vi "AnalogDemultiplexerV3_NI5771.vi"() -> ()   [LabVIEW 2012]
uses:
  <vilib>/Platform/TimedLoop/XDataNode/timing_clust.ctl
  <vilib>/Platform/TimedLoop/XDataNode/nitl_modes.ctl
  <vilib>/Platform/TimedLoop/XDataNode/wakeup.ctl
  <vilib>/rvi/FIFO/Fifo_Resource/nirvififoEmulationSetSize.vi
  <vilib>/rvi/DataTransferAndStorage/Container/Common/niFpgaContainerGetUniqueNameForEmu.vi
  <vilib>/rvi/eio/common/nirviEmuTemplateMethod_errors.vi
  <vilib>/rvi/Emulation/niFpgaSctlEmulationRegisterWithScheduler.vi
  <vilib>/rvi/errors/niFpgaSetErrorForExecOnDevCompSimple.vi
  <vilib>/rvi/eio/common/nirviEmuReportErrorAndStop.vi
  <vilib>/rvi/Emulation/niFpgaSctlEmulationFifoFullMgr.vi
  <vilib>/rvi/Emulation/niFpgaSctlEmulationResourceMgr.vi
  <vilib>/rvi/Emulation/niFpgaSctlEmulationScheduler.vi
  <vilib>/rvi/interface/RandomDataEmulation/nirviRandomDataFPGAFIFO.vi
  <vilib>/rvi/interface/RandomDataEmulation/niFpgaRandomDataHandleErrors.vi
  <vilib>/rvi/Emulation/niFpgaSctlEmulationGlobalWrite.vi
  <vilib>/Platform/TimedLoop/XDataNode/XDataNode.xnode
  <vilib>/rvi/DataTransferAndStorage/Container/XNode/niFpgaContainer.xnode
  <vilib>/rvi/FIFO/Fifo_Resource/nirvififoEmulationClear.vi
  <vilib>/eio/EIONode/EIONode.xnode
  <vilib>/rvi/FIFO/Fifo_Resource/nirvififoEmulationWrite.vi
  <vilib>/rvi/FIFO/Fifo_Resource/nirvififoEmulationRead.vi
  <vilib>/rvi/interface/RandomDataEmulation/nirviRandomDataFpgaReadWriteTemplate.vi
  <vilib>/Platform/TimedLoop/XDataNode/XDNodeRunTimeDep.lvlib
panel:
  out "Laser HIGH count per pixel":u16
  out "ToHostA2FIFO Overflow":bool
  out "ToHostA1FIFO Overflow":bool
  out "Pixel counter A2":u32
  out "Pixel counter A1":u32
  out "InterloopFIFO Overflow":bool
  in  "BaselineU8 Ch2":u8
  in  "BaselineU8 Ch1":u8
  out "InterloopFIFO timeout":bool
  in  "Clear Interloop FIFO":bool
  out "Acquiring":bool
  in  "Wait for trigger":bool
  in  "Acquire":bool
  in  "Requested pixels A2":u32=100000 caption="Requested pixels"
  in  "Acquire continuously":bool=TRUE
  in  "Requested pixels A1":u32=100000 caption="Requested pixels"
  in  "Samples per pixel":u16=10000 caption="Samples per pixel Acq"
  out "IO Module\\AI Over Range":bool
  in  "User Command Commit":bool
  in  "User Command":u8
  out "User Command Idle":bool
  out "User Command Status":u8
  in  "User Data 0":u16
  in  "User Data 1":u8
  out "PLL Locked":bool
  out "User Error":bool
  out "Configured?":bool
  # "5771 IO module configuration"
  # "Analog demultiplexer V3"
  # "Acquisition control"
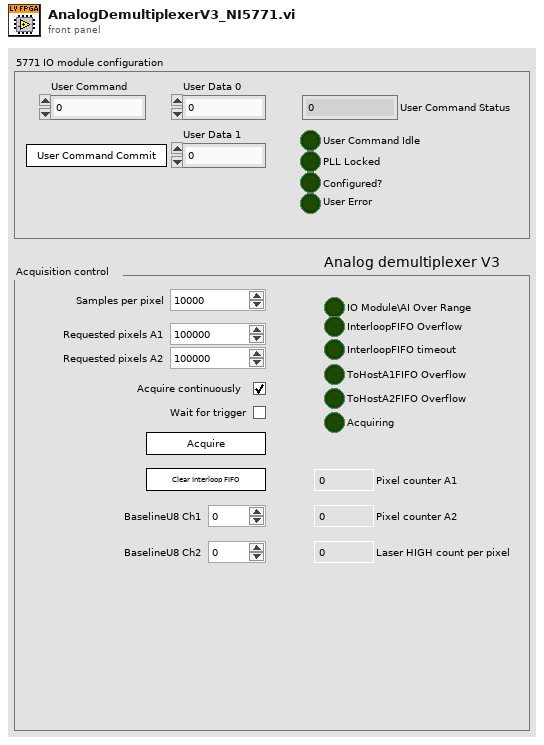
[diagram p1: front panel]
types:
  T1 = typedef "XDNodeRunTimeDep.lvlib/timing_clust.ctl" = cluster{"Expected End [f-1]":u64, "Actual End [f-1]":u64, "Finished Late? [f-1]":bool, "Expected End [i-1]":u64, "Actual End [i-1]":u64, "Finished Late? [i-1]":bool, "Expected Start [i]":u64, "Actual Start [i]":u64, "Expected Start [f]":u64, "Actual Start [f]":u64, "Source Name":string, "Structure Name":string, "Period":i64, "Deadline":i64, "Offset":i64, "Start":i64, "Priority":i32, "Timeout":i32, "Mode":T2, "Wakeup Reason":T3, "Error":errorcluster, "Source Type":string, "Secondary Source Type":string, "Global End Time":u64, "Global Start Time":u64, "Frame Duration":u64, "Iteration Duration":u64, "Assigned CPU":i32, "I/O Scan Engine Mode":u32}
  T2 = typedef "XDNodeRunTimeDep.lvlib/nitl_modes.ctl" = enum32{"No Change", "Process missed periods, maintain original phase", "Discard missed periods, maintain original phase", "Process missed periods, ignore original phase", "Discard missed periods, ignore original phase"}
  T3 = typedef "XDNodeRunTimeDep.lvlib/wakeup.ctl" = enum32{"Normal", "Aborted", "Asynchronous wakeup", "Timing source error", "Timed loop error", "Timeout"}
  T4 = cluster{"IO Module\\AI 0 Data N-7":u8, "IO Module\\AI 0 Data N-6":u8, "IO Module\\AI 0 Data N-5":u8, "IO Module\\AI 0 Data N-4":u8, "IO Module\\AI 0 Data N-3":u8, "IO Module\\AI 0 Data N-2":u8, "IO Module\\AI 0 Data N-1":u8, "IO Module\\AI 0 Data N":u8, "IO Module\\Synchronous Trigger Input":u8}
  T5 = cluster{"IO Module\\AI 1 Data N-7":u8, "IO Module\\AI 1 Data N-6":u8, "IO Module\\AI 1 Data N-5":u8, "IO Module\\AI 1 Data N-4":u8, "IO Module\\AI 1 Data N-3":u8, "IO Module\\AI 1 Data N-2":u8, "IO Module\\AI 1 Data N-1":u8, "IO Module\\AI 1 Data N":u8, "IO Module\\Synchronous Trigger Input":u8}
  T6 = cluster{"A1 Ch1":u32, "A1 Ch2":u32, "A2 Ch1":u32, "A2 Ch2":u32}
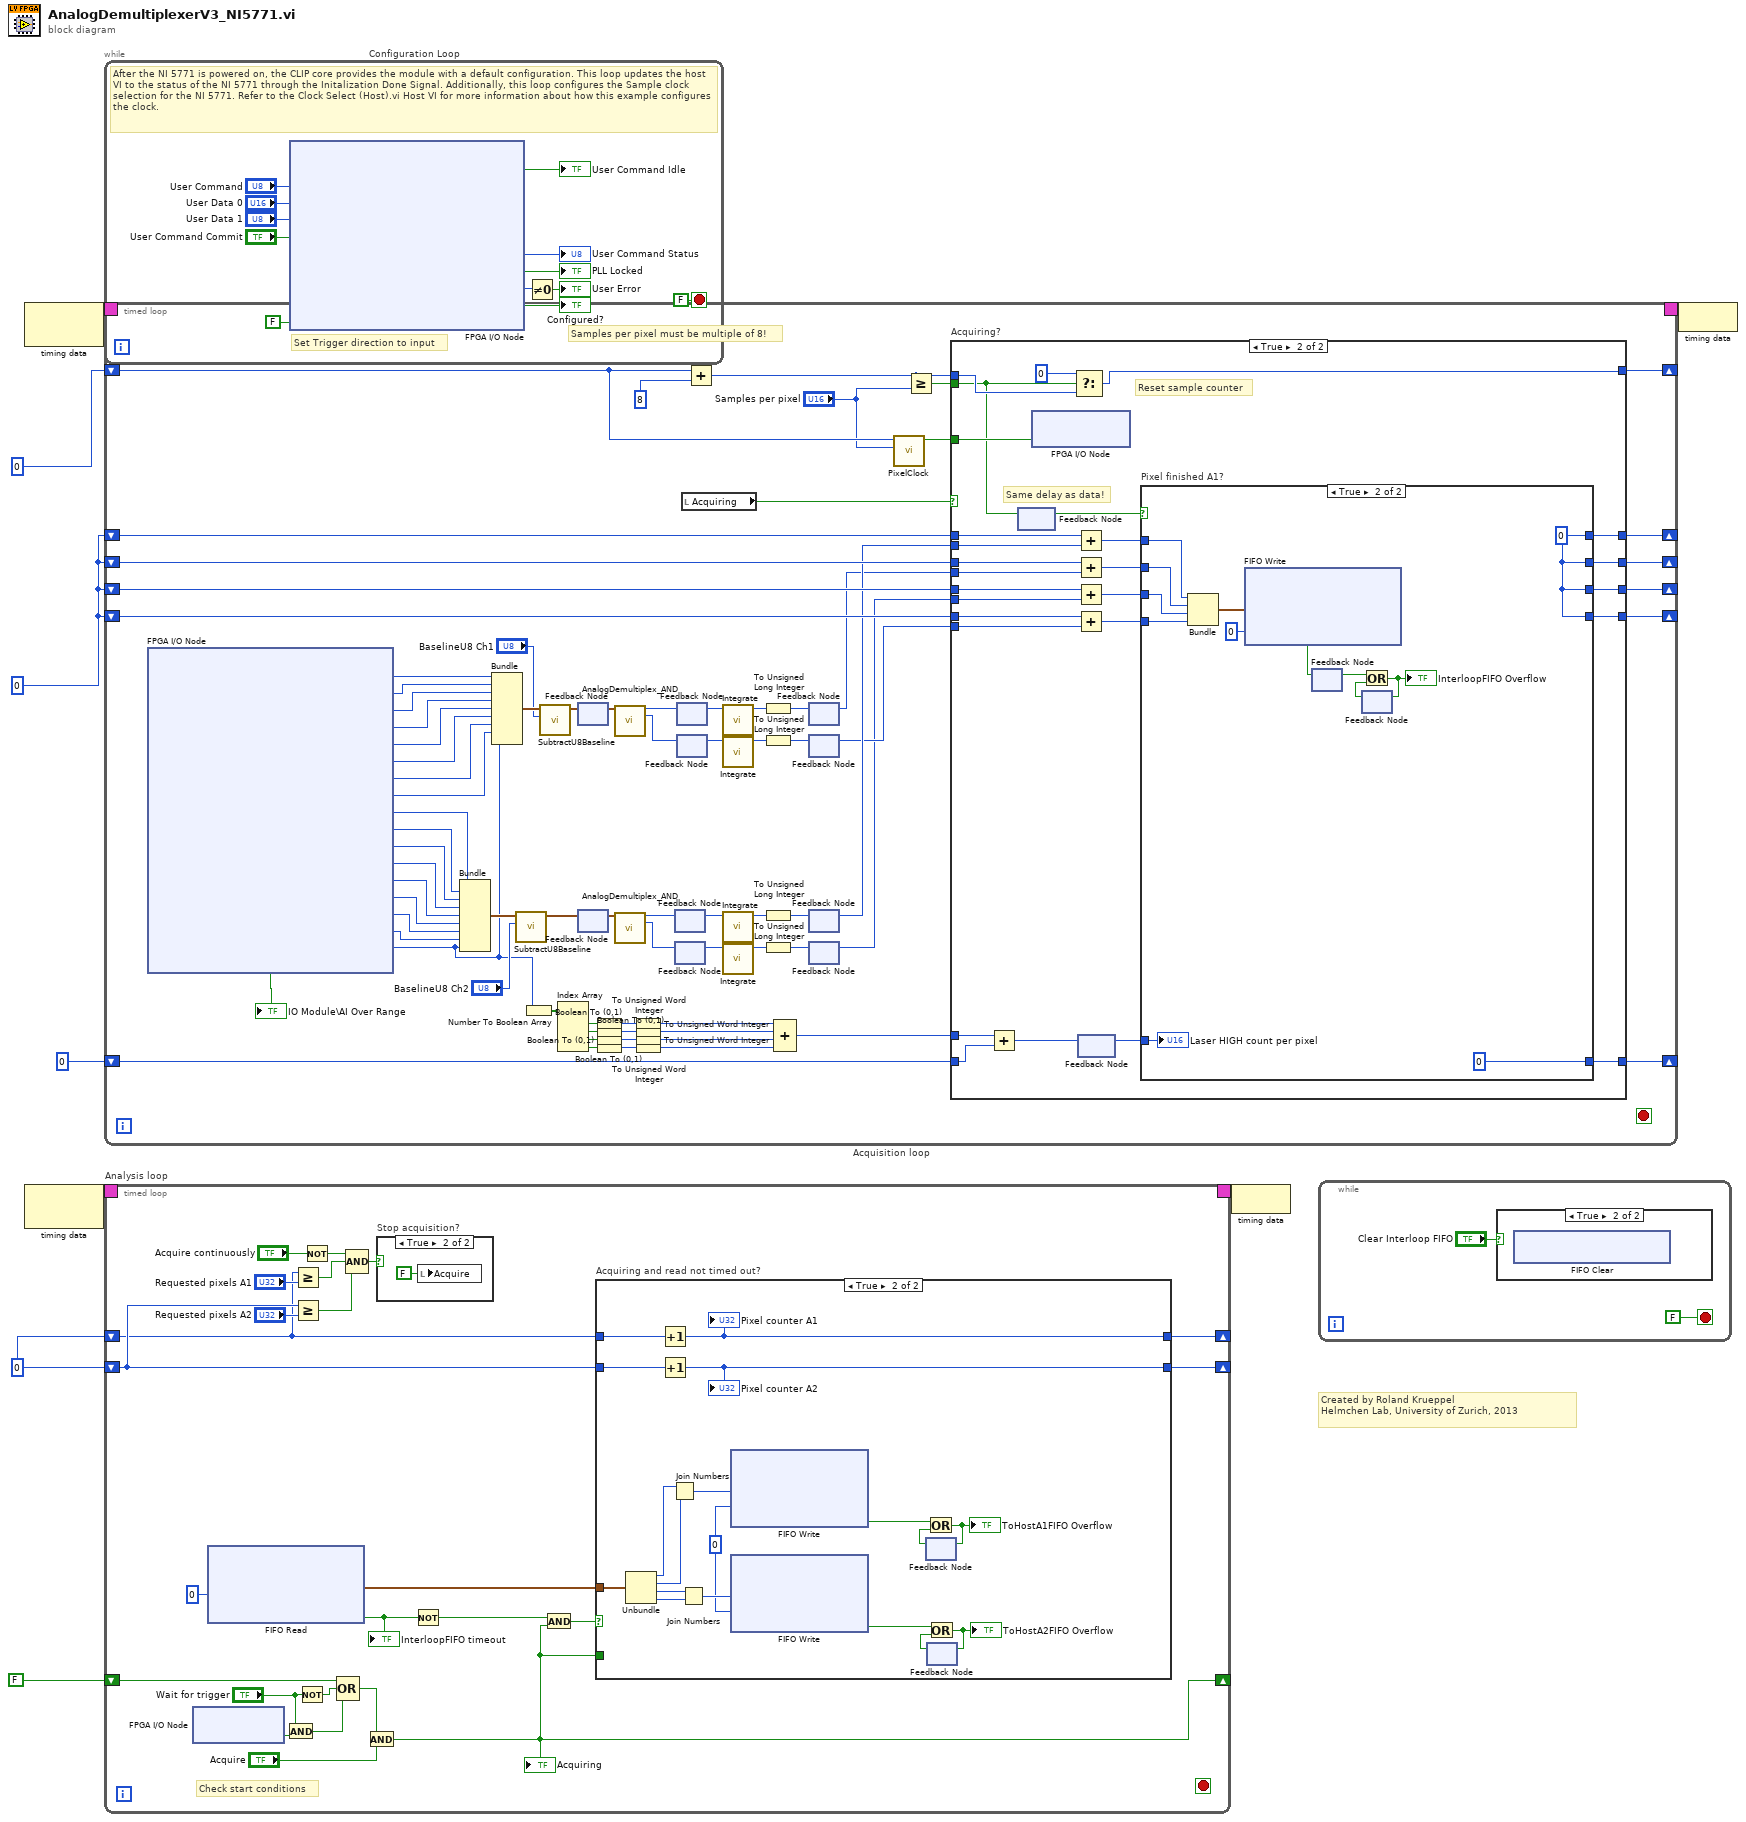
[diagram p0: block diagram]
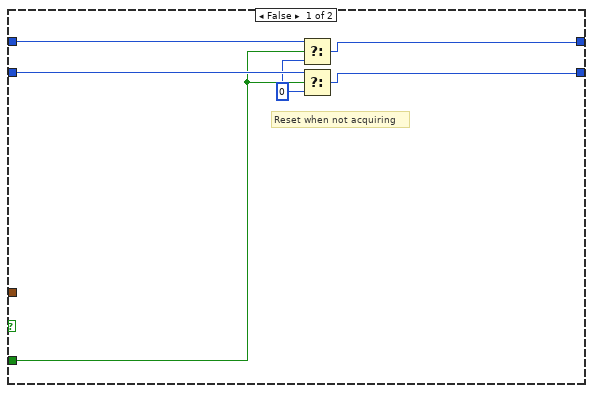
[diagram p3: hidden frame]
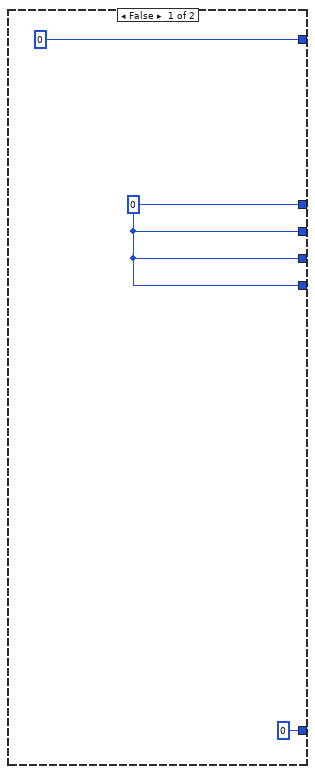
[diagram p5: hidden frame]
diagram:
  w2 = u32 0
  w3 = u32 0 ("Integrator out")
  # "Created by Roland Krueppel\nHelmchen Lab, University of Zurich, 2013"
  n1 = node-c288() -> (w9:T1)  [unwired: 1 in]
  n2 = node-c288() -> (w7:T1)  [unwired: 1 in]
  n3 = while "Configuration Loop" {
    stop <- FALSE stop-if-true
    # "Set Trigger direction to input"
    # "After the NI 5771 is powered on, the CLIP core provides the module with a default configuration. This loop updates the host VI to the status of the NI 5771 through the Initalization Done Signal. Additionally, this loop configures the Sample clock selection for the NI 5771. Refer to the Clock Select (Host).vi Host VI for more information about how this example configures the clock."
    n4 = xnode "FPGA I/O Node"("IO Module\\User Command"="User Command", "IO Module\\User Data 0"="User Data 0", "IO Module\\User Data 1"="User Data 1", "IO Module\\User Command Commit"="User Command Commit", "IO Module\\Trigger WE"=FALSE ("IO Module\\Trigger WE")) -> ("IO Module\\User Command Idle"=→"User Command Idle":bool, "IO Module\\User Command Status"=→"User Command Status":u8, "IO Module\\PLL Locked"=→"PLL Locked":bool, "IO Module\\User Error"=w14:u8, "IO Module\\Initialization Done"=→"Configured?":bool)  [unwired: 10 in, 10 out]
    n5 = Not Equal To 0?(x=w14) -> (x != 0?=→"User Error":bool)
  }
  n6 = timed-loop "Acquisition loop" {
    timing: w9 -> [_]
    timing-out: [_] -> w8
    shift-right: [w83] -> _
    shift-left: u16 0 -> [w70]
    shift-right: [w40] -> _
    shift-left: w2 -> [w49]
    shift-right: [w39] -> _
    shift-left: w2 -> [w48]
    shift-right: [w41] -> _
    shift-left: w2 -> [w50]
    shift-right: [w42] -> _
    shift-left: w2 -> [w51]
    shift-right: [w22] -> _
    shift-left: u16 0 -> [w23]
    stop <- _ stop-if-true
    # "Samples per pixel must be multiple of 8!"
    n7 = xnode "FPGA I/O Node"() -> ("IO Module\\AI 1 Data N-7"=w91:u8, "IO Module\\AI 1 Data N-6"=w90:u8, "IO Module\\AI 1 Data N-5"=w89:u8, "IO Module\\AI 1 Data N-4"=w88:u8, "IO Module\\AI 1 Data N-3"=w87:u8, "IO Module\\AI 1 Data N-2"=w86:u8, "IO Module\\AI 1 Data N-1"=w85:u8, "IO Module\\AI 1 Data N"=w84:u8, "IO Module\\AI 0 Data N-7"=w92:u8, "IO Module\\AI 0 Data N-6"=w93:u8, "IO Module\\AI 0 Data N-5"=w94:u8, "IO Module\\AI 0 Data N-4"=w95:u8, "IO Module\\AI 0 Data N-3"=w96:u8, "IO Module\\AI 0 Data N-2"=w97:u8, "IO Module\\AI 0 Data N-1"=w98:u8, "IO Module\\AI 0 Data N"=w99:u8, "IO Module\\Synchronous Trigger Input"=w38:u8, "IO Module\\AI Over Range"=→"IO Module\\AI Over Range":bool)  [unwired: 18 in, 18 out]
    n8 = Bundle("IO Module\\AI 0 Data N-7"=w92, "IO Module\\AI 0 Data N-6"=w93, "IO Module\\AI 0 Data N-5"=w94, "IO Module\\AI 0 Data N-4"=w95, "IO Module\\AI 0 Data N-3"=w96, "IO Module\\AI 0 Data N-2"=w97, "IO Module\\AI 0 Data N-1"=w98, "IO Module\\AI 0 Data N"=w99, "IO Module\\Synchronous Trigger Input"=w38) -> (w74:T4)  [unwired: 1 in]
    n9 = Bundle("IO Module\\AI 1 Data N-7"=w91, "IO Module\\AI 1 Data N-6"=w90, "IO Module\\AI 1 Data N-5"=w89, "IO Module\\AI 1 Data N-4"=w88, "IO Module\\AI 1 Data N-3"=w87, "IO Module\\AI 1 Data N-2"=w86, "IO Module\\AI 1 Data N-1"=w85, "IO Module\\AI 1 Data N"=w84, "IO Module\\Synchronous Trigger Input"=w38) -> (w77:T5)  [unwired: 1 in]
    n10 = call "SubtractU8Baseline.vi"("Baseline U8"="BaselineU8 Ch2", "Analog data cluster in"=w74) -> ("Analog data cluster out"=w73:T4)  [unwired: 9 in]
    n11 = Number To Boolean Array(number=w38) -> (Boolean array=w37:bool[])
    n12 = call "SubtractU8Baseline.vi"("Baseline U8"="BaselineU8 Ch1", "Analog data cluster in"=w77) -> ("Analog data cluster out"=w76:T4)  [unwired: 9 in]
    n13 = Index Array(array=w37) -> (element #1=w36:bool, element #2=w35:bool, element #3=w34:bool, element #4=w33:bool)  [unwired: 4 in]
    n14 = feedback-in #1(w76) -> ()
    n15 = feedback #1() -> (w82:T4)  [unwired: 1 in]
    n16 = feedback #2() -> (w78:T4)  [unwired: 1 in]
    n17 = feedback-in #2(w73) -> ()
    n18 = Boolean To (0,1)(Boolean=w36) -> (0, 1=w32:i16)
    n19 = Boolean To (0,1)(Boolean=w35) -> (0, 1=w31:i16)
    n20 = Boolean To (0,1)(Boolean=w34) -> (0, 1=w30:i16)
    n21 = Boolean To (0,1)(Boolean=w33) -> (0, 1=w29:i16)
    n22 = call "AnalogDemultiplex_AND.vi"("Analog data cluster"=w82) -> ("Data A1 out"=w67:u64, "Data A2 out"=w65:u64)  [unwired: 13 in]
    n23 = call "AnalogDemultiplex_AND.vi"("Analog data cluster"=w78) -> ("Data A1 out"=w63:u64, "Data A2 out"=w61:u64)  [unwired: 13 in]
    n24 = To Unsigned Word Integer(number=w32) -> (unsigned 16bit integer=w28:u16)
    n25 = To Unsigned Word Integer(number=w31) -> (unsigned 16bit integer=w27:u16)
    n26 = To Unsigned Word Integer(number=w30) -> (unsigned 16bit integer=w26:u16)
    n27 = To Unsigned Word Integer(number=w29) -> (unsigned 16bit integer=w25:u16)
    n28 = feedback #3() -> (w62:u64)  [unwired: 1 in]
    n29 = feedback-in #3(w63) -> ()
    n30 = feedback #4() -> (w60:u64)  [unwired: 1 in]
    n31 = feedback-in #4(w61) -> ()
    n32 = feedback-in #5(w67) -> ()
    n33 = feedback #5() -> (w66:u64)  [unwired: 1 in]
    n34 = feedback #6() -> (w64:u64)  [unwired: 1 in]
    n35 = feedback-in #6(w65) -> ()
    n36 = local read "Acquiring"() -> (w43:bool)
    n37 = Add(x=w70, y=u16 8) -> (x+y=w80:u16)
    n38 = call "Integrate.vi"("New samples in"=w66) -> ("Sum out"=w59:u16)  [unwired: 10 in]
    n39 = call "Integrate.vi"("New samples in"=w64) -> ("Sum out"=w58:u16)  [unwired: 10 in]
    n40 = call "Integrate.vi"("New samples in"=w62) -> ("Sum out"=w57:u16)  [unwired: 10 in]
    n41 = call "Integrate.vi"("New samples in"=w60) -> ("Sum out"=w56:u16)  [unwired: 10 in]
    n42 = To Unsigned Long Integer(number=w59) -> (unsigned 32bit integer=w55:u32)
    n43 = To Unsigned Long Integer(number=w58) -> (unsigned 32bit integer=w54:u32)
    n44 = To Unsigned Long Integer(number=w57) -> (unsigned 32bit integer=w53:u32)
    n45 = To Unsigned Long Integer(number=w56) -> (unsigned 32bit integer=w52:u32)
    n46 = Compound Arithmetic op=unknown(w28, w27, w26, w25) -> (w24:u16)
    n47 = feedback #7() -> (w46:u32)  [unwired: 1 in]
    n48 = feedback-in #7(w55) -> ()
    n49 = feedback #8() -> (w45:u32)  [unwired: 1 in]
    n50 = feedback-in #8(w54) -> ()
    n51 = feedback #9() -> (w47:u32)  [unwired: 1 in]
    n52 = feedback-in #9(w53) -> ()
    n53 = feedback #10() -> (w44:u32)  [unwired: 1 in]
    n54 = feedback-in #10(w52) -> ()
    n55 = call "PixelClock.vi"("Samples per pixel"="Samples per pixel", "Sample counter"=w70) -> ("Pixel clock"=w68:bool)  [unwired: 9 in]
    n56 = Greater Or Equal?(x=w80, y="Samples per pixel") -> (x >= y?=w79:bool)
    n57 = case "Acquiring?" shown="True" w43 {
      tunnel: [u16 0 ("t") w129] -> w83
      tunnel: w80 -> [_ w128]
      tunnel: w79 -> [_ w113]
      tunnel: w68 -> [_ w118]
      tunnel: w51 -> [_ w127]
      tunnel: w50 -> [_ w126]
      tunnel: w49 -> [_ w125]
      tunnel: w48 -> [_ w124]
      tunnel: w47 -> [_ w123]
      tunnel: w46 -> [_ w122]
      tunnel: w45 -> [_ w121]
      tunnel: w44 -> [_ w120]
      tunnel: [w101 w111] -> w42
      tunnel: [w101 w110] -> w41
      tunnel: [w101 w109] -> w40
      tunnel: [w101 w108] -> w39
      tunnel: w24 -> [_ w107]
      tunnel: w23 -> [_ w106]
      tunnel: [u16 0 w103] -> w22
      frame False {
        w101 = u32 0
      }
      frame True {
        # "Same delay as data!"
        # "Reset sample counter"
        n58 = Add(x=w107, y=w106) -> (x+y=w105:u16)
        n59 = feedback #11() -> (w112:bool)  [unwired: 1 in]
        n60 = feedback-in #11(w113) -> ()
        n61 = xnode "FPGA I/O Node"("Pixel clock"=w118) -> ()  [unwired: 1 in, 1 out]
        n62 = Select(t=u16 0, s=w113, f=w128) -> (s? t:f=w129:u16)
        n63 = Add(x=w127, y=w123) -> (x+y=w117:u32)
        n64 = Add(x=w126, y=w122) -> (x+y=w116:u32)
        n65 = Add(x=w125, y=w120) -> (x+y=w115:u32)
        n66 = Add(x=w124, y=w121) -> (x+y=w114:u32)
        n67 = feedback-in #12(w105) -> ()
        n68 = feedback #12() -> (w104:u16)  [unwired: 1 in]
        n69 = case "Pixel finished A1?" shown="True" w112 {
          tunnel: w117 -> [w134 w147]
          tunnel: w116 -> [w133 w146]
          tunnel: w115 -> [w132 w145]
          tunnel: w114 -> [w131 w144]
          tunnel: [w134 w137] -> w111
          tunnel: [w133 w137] -> w110
          tunnel: [w132 w137] -> w109
          tunnel: [w131 w137] -> w108
          tunnel: w104 -> [w130 w136]
          tunnel: [w130 u16 0] -> w103
          frame False {
          }
          frame True {
            w137 = u32 0
            n70 = Bundle(w147, w146, w145, w144) -> (w143:cluster{u32, u32, u32, u32})  [unwired: 1 in]
            n71 = xnode ("FIFO Write")("Element"=w143, "Timeout"=0) -> ("Timed Out?"=w138:bool)  [unwired: 1 in, 1 out]
            n72 = feedback #13() -> (w139:bool)  [unwired: 1 in]
            n73 = feedback-in #13(w138) -> ()
            n74 = feedback #14() -> (w140:bool)  [unwired: 1 in]
            n75 = Or(x=w139, y=w140) -> (x .or. y?=w141:bool)
            "InterloopFIFO Overflow" <- w141
            n76 = feedback-in #14(w141) -> ()
            "Laser HIGH count per pixel" <- w136
          }
        }
      }
    }
  }
  n77 = timed-loop "Analysis loop" {
    timing: w7 -> [_]
    timing-out: [_] -> w6
    shift-right: [w150] -> _
    shift-left: FALSE -> [w160]
    shift-right: [w153] -> _
    shift-left: w3 -> [w154]
    shift-right: [w152] -> _
    shift-left: w3 -> [w155]
    stop <- _ stop-if-true
    # "Check start conditions"
    n78 = xnode "FPGA I/O Node"() -> ("TriggerIn"=w165:bool)  [unwired: 1 in, 1 out]
    n79 = xnode ("FIFO Read")("Timeout"=0) -> ("Element"=w151:T6, "Timed Out?"=w157:bool)  [unwired: 1 in, 1 out]
    "InterloopFIFO timeout" <- w157
    n80 = And(x="Wait for trigger", y=w165) -> (x .and. y?=w162:bool)
    n81 = Greater Or Equal?(x=w154, y="Requested pixels A1") -> (x >= y?=w168:bool)
    n82 = Greater Or Equal?(x=w155, y="Requested pixels A2") -> (x >= y?=w167:bool)
    n83 = Not(x="Wait for trigger") -> (.not. x?=w163:bool)
    n84 = Not(x="Acquire continuously") -> (.not. x?=w169:bool)
    n85 = Compound Arithmetic op=OR(w160, w163, w162) -> (w161:bool)
    n86 = Compound Arithmetic op=AND(w169, w168, w167) -> (w159:bool)
    n87 = And(x=w161, y="Acquire") -> (x .and. y?=w150:bool)
    "Acquiring" <- w150
    n88 = case "Stop acquisition?" shown="True" w159 {
      frame False {
      }
      frame True {
        n89 = local write "Acquire"(FALSE ("Acquire")) -> ()
      }
    }
    n90 = Not(x=w157) -> (.not. x?=w156:bool)
    n91 = And(x=w156, y=w150) -> (x .and. y?=w158:bool)
    n92 = case "Acquiring and read not timed out?" shown="True" w158 {
      tunnel: w155 -> [w177 w196]
      tunnel: w154 -> [w179 w197]
      tunnel: [w178 w194] -> w153
      tunnel: [w176 w195] -> w152
      tunnel: w151 -> [_ w193]
      tunnel: w150 -> [w175 _]
      frame False {
        w174 = u32 0 ("f")
        # "Reset when not acquiring"
        n93 = Select(t=w179, s=w175, f=w174) -> (s? t:f=w178:u32)
        n94 = Select(t=w177, s=w175, f=w174) -> (s? t:f=w176:u32)
      }
      frame True {
        w186 = 0 ("Timeout")
        n95 = Unbundle(w193) -> ("A1 Ch1"=w192:u32, "A1 Ch2"=w191:u32, "A2 Ch1"=w189:u32, "A2 Ch2"=w188:u32)
        n96 = Increment(x=w197) -> (x+1=w194:u32)
        "Pixel counter A1" <- w194
        n97 = Increment(x=w196) -> (x+1=w195:u32)
        "Pixel counter A2" <- w195
        n98 = Join Numbers(hi=w192, lo=w191) -> ((hi.lo)=w190:u64)
        n99 = Join Numbers(hi=w189, lo=w188) -> ((hi.lo)=w187:u64)
        n100 = xnode ("FIFO Write")("Element"=w190, "Timeout"=w186) -> ("Timed Out?"=w184:bool)  [unwired: 1 in, 1 out]
        n101 = xnode ("FIFO Write")("Element"=w187, "Timeout"=w186) -> ("Timed Out?"=w180:bool)  [unwired: 1 in, 1 out]
        n102 = feedback #15() -> (w183:bool)  [unwired: 1 in]
        n103 = Or(x=w184, y=w183) -> (x .or. y?=w185:bool)
        "ToHostA1FIFO Overflow" <- w185
        n104 = feedback-in #15(w185) -> ()
        n105 = feedback #16() -> (w181:bool)  [unwired: 1 in]
        n106 = Or(x=w180, y=w181) -> (x .or. y?=w182:bool)
        "ToHostA2FIFO Overflow" <- w182
        n107 = feedback-in #16(w182) -> ()
      }
    }
  }
  n108 = node-c288(w6) -> ()
  n109 = while {
    stop <- FALSE stop-if-true
    n110 = case shown="True" "Clear Interloop FIFO" {
      frame False {
      }
      frame True {
        n111 = xnode ("FIFO Clear")() -> ()  [unwired: 1 in, 1 out]
      }
    }
  }
  n112 = node-c288(w8) -> ()
